vi "LcWebView_Create.vi"(0 "reference in":refnum<class "LcWebView.lvclass">, 1 "Webview container":refnum<k24>(container), 2 "User Data Folder":path, 5 "Error In":errorcluster) -> (12 "BrowserProcessId":u32, 13 "User Data Folder":path, 14 "reference out":refnum<class "LcWebView.lvclass">, 15 "Status":i32(ring)=5 items=["Created", "WaitingForActivation", "WaitingToRun", "Running", "WaitingForChildrenToComplete", "RanToCompletion", "Canceled", "Faulted"], 16 "Status Message":string, 17 "Initialise Loops":i32=1, 18 "Reinstall Runtime":bool, 19 "Error Out":errorcluster)   [LabVIEW 2019, in "LcWebView.lvclass"]
uses:
  LcWebView.lvclass
  C:/Projects/WebView2/LcWebView/data/Microsoft.Web.WebView2.WinForms.dll
  ctrls/ErrorCode.ctl
  C:/Projects/WebView2/LcWebView/data/Microsoft.Web.WebView2.Core.dll
  SourceChangeEvent.vi
  ctrls/PlotType.ctl
  ctrls/PlotRef.ctl
  ctrls/PlotMap.ctl
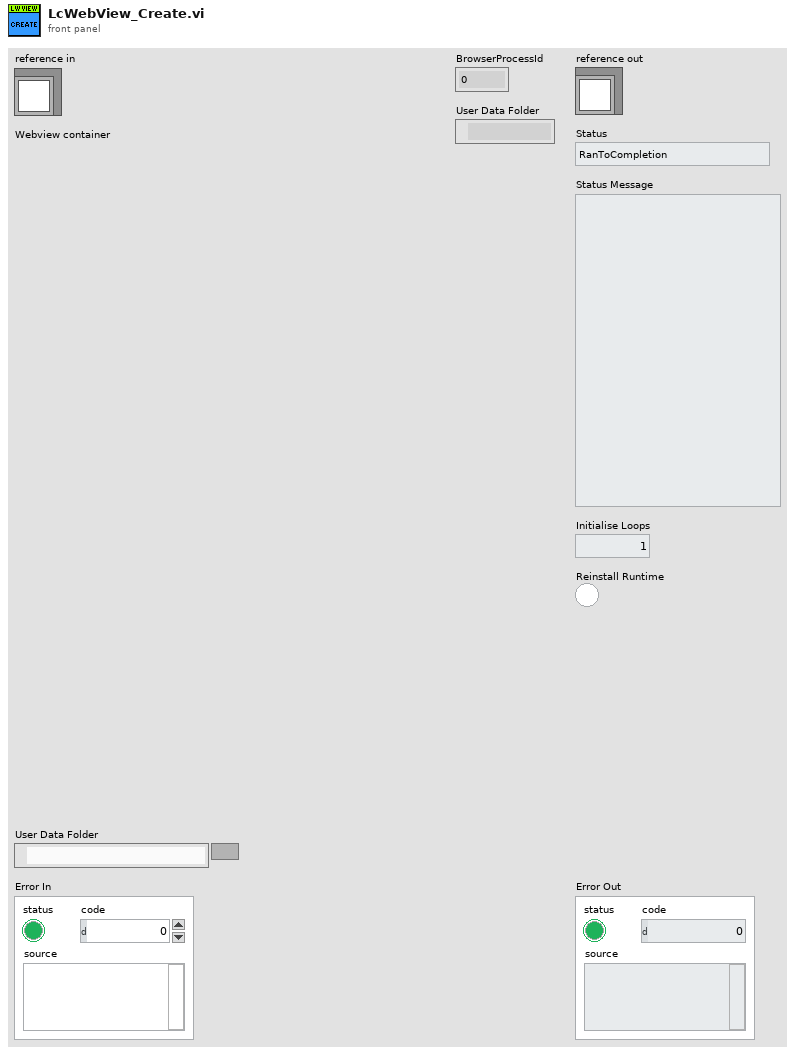
[diagram p1: front panel]
types:
  T1 = typedef "LcWebView.lvclass/PlotMap.ctl" = map{string, T2}
  T2 = typedef "LcWebView.lvclass/PlotRef.ctl" = cluster{"PlotType":T3, "PlotTemplate":string}
  T3 = typedef "LcWebView.lvclass/PlotType.ctl" = enum16{"bar", "line", "pie"}
  T4 = typedef "LcWebView.lvclass/ErrorCode.ctl" = enum16{"Runtime engine is not installed or incompatible", "User Data Folder cannot be set", "Others"}
  T5 = typedef "LcWebView.lvclass/ObjectAttributes.ctl" = cluster{"WebView Container":refnum<k24>, "CoreWebViewRef":refnum<k24>, "Status":i32, "Status Message":string, "User Data Folder":path, "DynamicEvents":T6, "BrowserProcessId":u32, "PlotMap":T7, "PlotType":T3}
  T6 = typedef "LcWebView.lvclass/WebViewDynamicEvents.ctl" = cluster{"Event Registration Ref":refnum<event-registration>, "Source event":refnum<user-event>}
  T7 = typedef "PlotMap.ctl" = map{string, T8}
  T8 = typedef "PlotRef.ctl" = cluster{"PlotType":T3, "PlotTemplate":string}
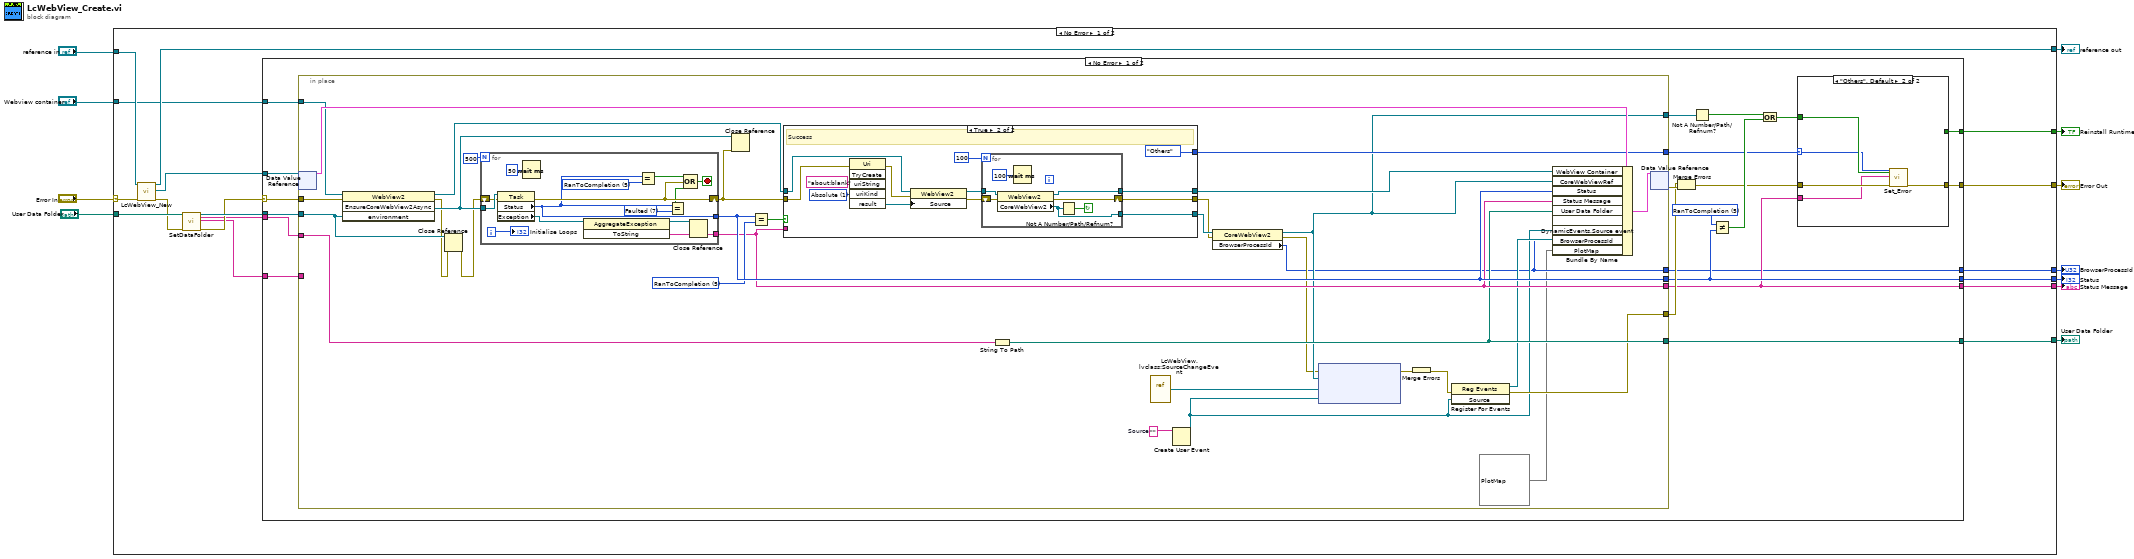
[diagram p0: block diagram]
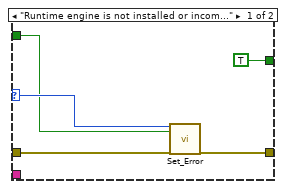
[diagram p2: hidden frame]
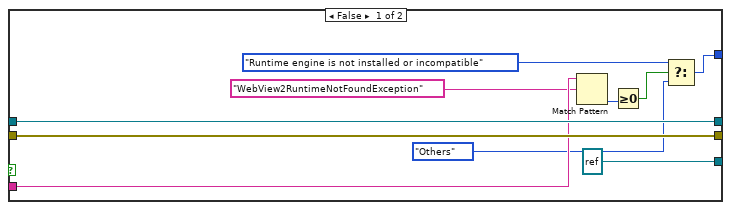
[diagram p3: hidden frame]
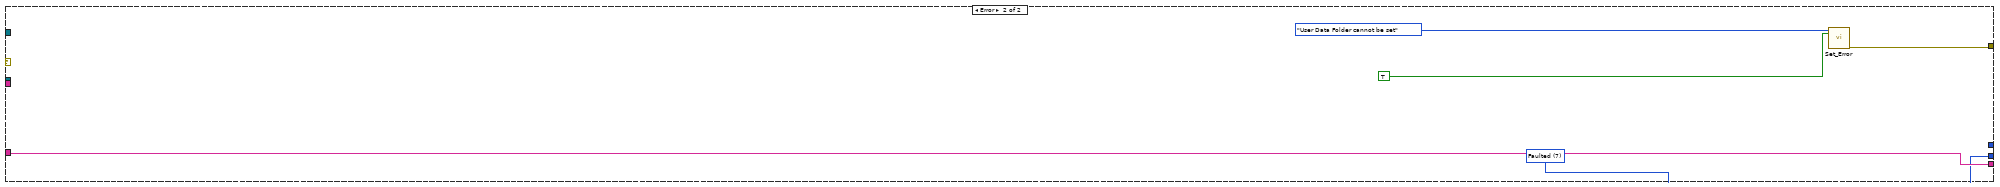
[diagram p4: hidden frame]
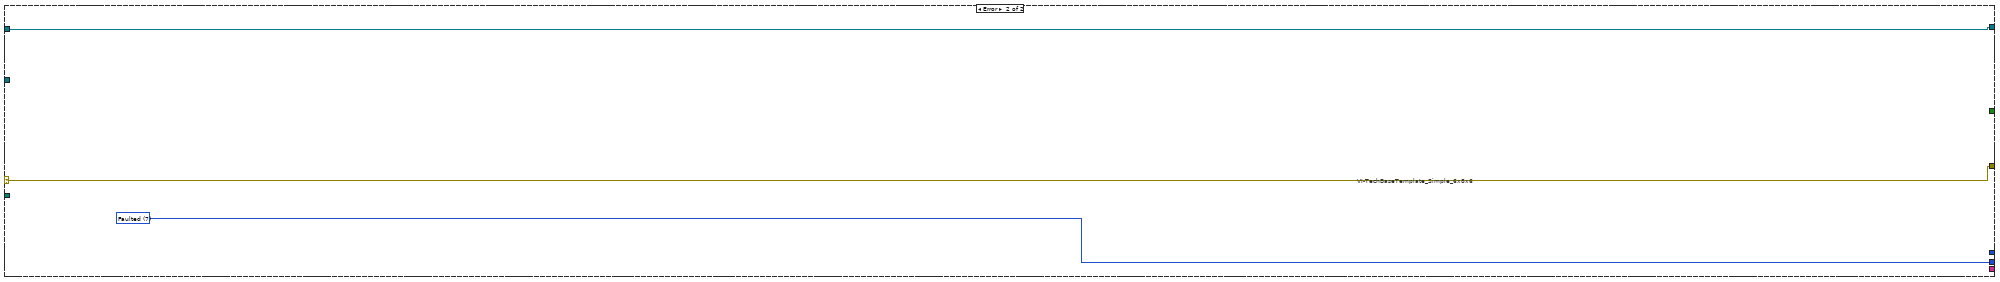
[diagram p5: hidden frame]
diagram:
  n1 = case shown="No Error" "Error In" {
    selector: "Error In" -> [w20 w143]
    tunnel: [w23 w143] -> w10
    tunnel: "reference in" -> [w28 w142]
    tunnel: [w27 w142] -> w8
    tunnel: [w25 w141] -> w7
    tunnel: [w22 _] -> w6
    tunnel: "Webview container" -> [w24 _]
    tunnel: [w21 _] -> w4
    tunnel: "User Data Folder" -> [w19 _]
    tunnel: [w13 _] -> w2
    tunnel: [w12 _] -> w1
    frame No Error {
      n2 = call "LcWebView_New.vi"("reference in"=w28, "error in (no error)"=w20) -> ("reference out"=w27:refnum<class "LcWebView.lvclass">, "DVRRefOut"=w26:refnum<data-value>, "error out"=w16:errorcluster)  [unwired: 14 in, 1 out]
      n3 = call "SetDataFolder.vi"("User Data Folder"=w19, "error in (no error)"=w16) -> ("Environment"=w18:refnum<k24>, "UserDataFolder"=w14:string, "Error Message"=w15:string, "error out"=w17:errorcluster)  [unwired: 14 in]
      n4 = case shown="No Error" w17 {
        selector: w17 -> [w33 _]
        tunnel: w26 -> [w48 _]
        tunnel: [w46 w137] -> w25
        tunnel: w24 -> [w43 _]
        tunnel: [w38 w140] -> w23
        tunnel: [w36 w139] -> w22
        tunnel: [w35 _] -> w21
        tunnel: w18 -> [w34 _]
        tunnel: w15 -> [w32 w139]
        tunnel: w14 -> [w31 _]
        tunnel: [w30 _] -> w13
        tunnel: [w29 _] -> w12
        frame No Error {
          w45 = 5 items=["Created", "WaitingForActivation", "WaitingToRun", "Running", "WaitingForChildrenToComplete", "RanToCompletion", "Canceled", "Faulted"] ("Status")
          n5 = in-place {
            in-place-border: w43 -> [w81]
            in-place-border: [w88] -> w46
            in-place-border: [w83] -> w36
            in-place-border: [w68] -> w47
            in-place-border: [w64] -> w42
            in-place-border: [w82] -> w37
            in-place-border: w34 -> [w75]
            in-place-border: w33 -> [w78]
            in-place-border: w32 -> [_]
            in-place-border: w31 -> [w77]
            in-place-border: [w76] -> w30
            in-place-border: [w61] -> w29
            w72 = ""  # Source
            w87 = 5 items=["Created", "WaitingForActivation", "WaitingToRun", "Running", "WaitingForChildrenToComplete", "RanToCompletion", "Canceled", "Faulted"] ("Status")
            n6 = in-place-dvr #1(w48) -> (w90:T5)  [unwired: 1 out]
            n7 = invoke class="WebView2" method="EnsureCoreWebView2Async"(reference=w81, error in=w78, "environment"=w75) -> (reference out=w79:refnum<k24>, error out=w74:errorcluster, "EnsureCoreWebView2Async"=w85:refnum<k24>)  [unwired: 1 in, 1 out]
            n8 = Close Reference(reference=w75, error in (no error)=w74) -> (error out=w73:errorcluster)
            n9 = for {
              N: 500 -> [_]
              tunnel: w85 -> [w135]
              shift-right: [w128] -> w84
              shift-left: w73 -> [w134]
              tunnel: [w125] -> w88
              tunnel: [w131] -> w83
              i -> [w123]
              stop <- w126 stop-if-true
              w130 = 5 items=["Created", "WaitingForActivation", "WaitingToRun", "Running", "WaitingForChildrenToComplete", "RanToCompletion", "Canceled", "Faulted"] ("Status")
              w132 = 7 items=["Created", "WaitingForActivation", "WaitingToRun", "Running", "WaitingForChildrenToComplete", "RanToCompletion", "Canceled", "Faulted"] ("Status")
              n10 = property class="Task"(reference=w135, error in=w134) -> (error out=w128:errorcluster, "Status"=w125:i32, "Exception"=w133:refnum<k24>)  [unwired: 1 out]
              n11 = Wait (ms)(milliseconds to wait=u32 50) -> ()  [unwired: 1 out]
              n12 = invoke class="AggregateException" method="ToString"(reference=w133) -> (reference out=w124:refnum<k24>, "ToString"=w131:string)  [unwired: 2 in, 1 out]
              n13 = Equal?(x=w125, y=w130) -> (x = y?=w129:bool)
              n14 = Equal?(x=w125, y=w132) -> (x = y?=w127:bool)
              n15 = Compound Arithmetic op=OR(w129, w128, w127) -> (w126:bool)
              n16 = Close Reference(reference=w124) -> ()  [unwired: 1 in, 1 out]
              "Initialise Loops" <- w123
            }
            n17 = Close Reference(reference=w85, error in (no error)=w84) -> ()  [unwired: 1 out]
            n18 = Equal?(x=w88, y=w87) -> (x = y?=w86:bool)
            n19 = case shown="True" w86 {
              tunnel: w84 -> [w99 w106]
              tunnel: [w101 w114] -> w80
              tunnel: [refnum<k24> refnum ("CoreWebView2") w113] -> w65
              tunnel: [w99 w112] -> w63
              tunnel: w79 -> [w101 w105]
              tunnel: w83 -> [w98 _]
              tunnel: [w92 ErrorCode."Others" ("f")] -> w82
              frame False {
                n20 = Match Pattern(string=w98, regular expression="WebView2RuntimeNotFoundException") -> (offset past match=w96:i32)  [unwired: 1 in, 3 out]
                n21 = Greater Or Equal To 0?(x=w96) -> (x >= 0?=w95:bool)
                n22 = Select(t=ErrorCode."Runtime engine is not installed or incompatible" ("CustomErrors"), s=w95, f=ErrorCode."Others") -> (s? t:f=w92:T4)
              }
              frame True {
                w108 = 1 items=["RelativeOrAbsolute", "Absolute", "Relative"] ("uriKind")
                # "Success"
                n23 = invoke class="Uri" method="TryCreate"(error in=w106, "uriString"="about:blank", "uriKind"=w108) -> (error out=w103:errorcluster, "result"=w107:refnum<k24>)  [unwired: 3 in, 4 out]
                n24 = property class="WebView2"(reference=w105, error in=w103, "Source"=w107) -> (reference out=w104:refnum<k24>, error out=w102:errorcluster)
                n25 = for {
                  N: 100 -> [_]
                  tunnel: w104 -> [w121]
                  shift-right: [w118] -> w112
                  shift-left: w102 -> [w119]
                  tunnel: [w116] -> w113
                  tunnel: [w115] -> w114
                  stop <- w117 continue-if-true
                  n26 = property class="WebView2"(reference=w121, error in=w119) -> (reference out=w115:refnum<k24>, error out=w118:errorcluster, "CoreWebView2"=w116:refnum<k24>)
                  n27 = Wait (ms)(milliseconds to wait=u32 100) -> ()  [unwired: 1 out]
                  n28 = Not A Number/Path/Refnum?(number/path/refnum=w116) -> (NaN/Path/Refnum?=w117:bool)
                }
              }
            }
            n29 = String To Path(string=w77) -> (path=w76:path)
            n30 = vi-ref "LcWebView.lvclass:SourceChangeEvent.vi"() -> ("vi reference"=w66:refnum<vi>)
            n31 = Create User Event(user event datatype=w72) -> (user event=w67:refnum<user-event>)  [unwired: 1 in, 1 out]
            n32 = property class="CoreWebView2"(reference=w65, error in=w63) -> (reference out=w64:refnum<k24>, error out=w62:errorcluster, "BrowserProcessId"=w61:u32)
            n33 = node(w62, w64, w66, w67) -> (w71:errorcluster)  [unwired: 1 in, 1 out]
            n34 = Merge Errors(w71) -> (w69:errorcluster)
            n35 = register-events(error in=w69, w67) -> (reference out=w70:refnum<event-registration>, error out=w68:errorcluster)  [unwired: 1 in]
            n36 = Bundle By Name(cluster=w90, "WebView Container"=w80, "CoreWebViewRef"=w64, "Status"=w88, "Status Message"=w83, "User Data Folder"=w76, "DynamicEvents.Event Registration Ref"=w70, "DynamicEvents.Source event"=w67, "BrowserProcessId"=w61, "PlotMap"=T1 {}) -> (w91:T5)
            n37 = in-place-dvr #1(w91) -> (w49:errorcluster)  [unwired: 1 out]
          }
          n38 = Merge Errors(w47, w49) -> (w40:errorcluster)
          n39 = Not A Number/Path/Refnum?(number/path/refnum=w42) -> (NaN/Path/Refnum?=w41:bool)
          n40 = Not Equal?(x=w45, y=w46) -> (x != y?=w44:bool)
          n41 = Compound Arithmetic op=OR(w41, w44) -> (w39:bool)
          n42 = case shown="\"Others\", Default" w37 {
            selector: w37 -> [w52 w56]
            tunnel: w40 -> [w54 w59]
            tunnel: w39 -> [w51 w58]
            tunnel: [w53 w57] -> w38
            tunnel: w36 -> [_ w55]
            tunnel: [TRUE _] -> w35
            frame "Runtime engine is not installed or incompatible" {
              n43 = call "Set_Error.vi"("CustomErrors"=w52, "SetError(True)"=w51, "error in (no error)"=w54) -> ("error out"=w53:errorcluster)  [unwired: 16 in]
            }
            frame "Others", Default {
              n44 = call "Set_Error.vi"("CustomErrors"=w56, "SetError(True)"=w58, "Description"=w55, "error in (no error)"=w59) -> ("error out"=w57:errorcluster)  [unwired: 15 in]
            }
          }
        }
        frame Error {
          w137 = 7 items=["Created", "WaitingForActivation", "WaitingToRun", "Running", "WaitingForChildrenToComplete", "RanToCompletion", "Canceled", "Faulted"] ("Status")
          n45 = call "Set_Error.vi"("CustomErrors"=ErrorCode."User Data Folder cannot be set", "SetError(True)"=TRUE) -> ("error out"=w140:errorcluster)  [unwired: 17 in]
        }
      }
    }
    frame Error {
      w141 = 7 items=["Created", "WaitingForActivation", "WaitingToRun", "Running", "WaitingForChildrenToComplete", "RanToCompletion", "Canceled", "Faulted"] ("Status")
      # "VI-TechBaseTemplate_Simple_6x8x6"
    }
  }
  "Error Out" <- w10
  "reference out" <- w8
  "Status" <- w7
  "Status Message" <- w6
  "Reinstall Runtime" <- w4
  "User Data Folder" <- w2
  "BrowserProcessId" <- w1
